vi "Stringlength.vi"() -> ()   [LabVIEW 2019]
panel:
  out "length":i32
  in  "str":string="Pomogranate"
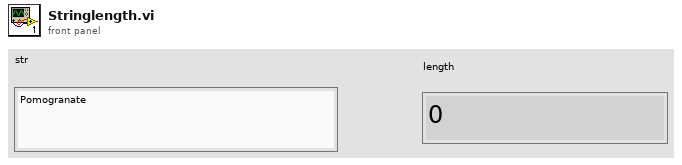
[diagram p1: front panel]
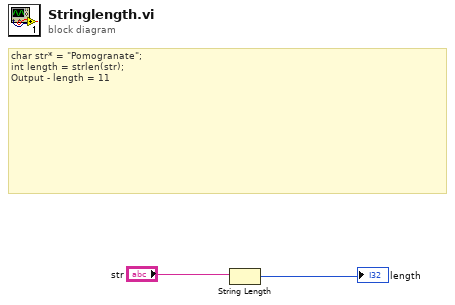
[diagram p0: block diagram]
diagram:
  # "char str* = \"Pomogranate\";\nint length = strlen(str);\nOutput - length = 11"
  n1 = String Length(string="str") -> (length=→"length":i32)
